vi "set power.vi"(8 "error in (no error)":errorcluster, 11 "Cobolt in":refnum<class "Cobolt.lvclass">) -> (0 "error out":errorcluster, 3 "Cobolt out":refnum<class "Cobolt.lvclass">)   [LabVIEW 2012, in "Cobolt.lvclass"]
uses:
  Cobolt.lvclass
  CoboltLaserDrivers_Public_LV2012/CoboltLaser_Controls/ExpectedResponseType.ctl
  Cobolt.lvclass/Cobolt.ctl
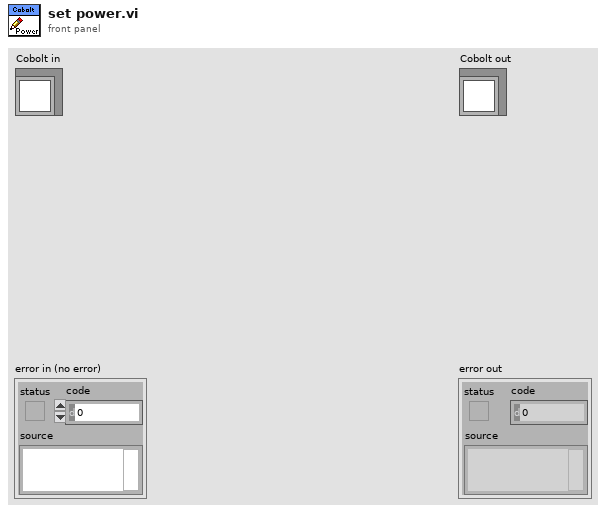
[diagram p1: front panel]
types:
  T1 = typedef "Cobolt.lvclass/ExpectedResponseType.ctl" = u16
  T2 = typedef "Cobolt.lvclass/powermW.ctl" = dbl[unit]
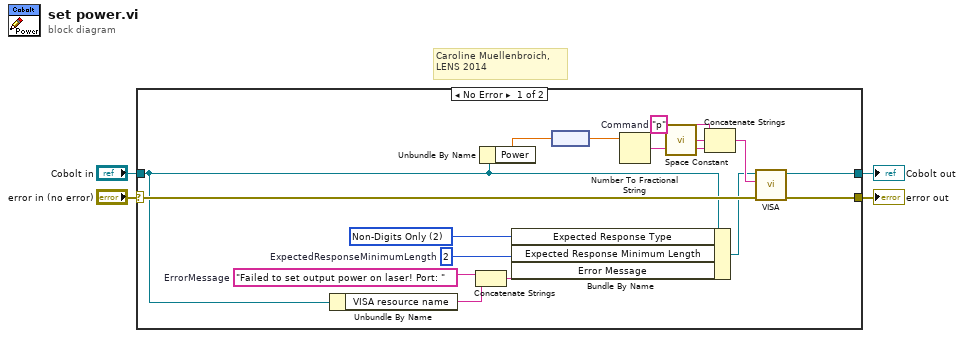
[diagram p0: block diagram]
diagram:
  # "Caroline Muellenbroich, \nLENS 2014"
  n1 = case shown="No Error" "error in (no error)" {
    selector: "error in (no error)" -> [w17 w22]
    tunnel: [w6 w22] -> w3
    tunnel: [w5 w21] -> w1
    tunnel: "Cobolt in" -> [w9 w21]
    frame No Error {
      w10 = T1 2 items=["Any", "Digits Only", "Non-Digits Only"] ("ExpectedResponseType")
      w14 = 2  # ExpectedResponseMinimumLength
      w12 = "Failed to set output power on laser! Port: "  # ErrorMessage
      w18 = "p"  # Command
      n2 = Unbundle By Name(w9) -> ("VISA resource name"=w13:string)
      n3 = Concatenate Strings(w12, w13) -> (w11:string)
      n4 = Unbundle By Name(w9) -> ("Power"=w7:T2)
      n5 = Bundle By Name(cluster=w9, "Expected Response Type"=w10, "Expected Response Minimum Length"=w14, "Error Message"=w11) -> (w15:refnum<class "Cobolt.lvclass">)
      n6 = node(w7) -> (w8:dbl)
      n7 = Number To Fractional String(number=w8) -> (F-format string=w20:string)  [unwired: 3 in]
      n8 = call <vilib>:"Space Constant.vi"() -> ("String"=w19:string)
      n9 = Concatenate Strings(w18, w19, w20) -> (w16:string)
      n10 = call-dynamic "VISA.vi"("error in (no error)"=w17, "string to write"=w16, "Cobolt in"=w15) -> ("error out"=w6:errorcluster, "Cobolt out"=w5:refnum<class "Cobolt.lvclass">)  [unwired: 6 in, 1 out]
    }
    frame Error {
    }
  }
  "error out" <- w3
  "Cobolt out" <- w1
